vi "密码到期.vi"() -> ()   [LabVIEW 2016]
panel:
  out "密码生效":bool
  out "到期了":bool
  in  "密码输入":string
  in  "停止":bool
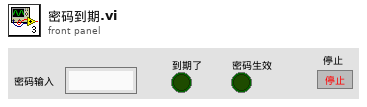
[diagram p1: front panel]
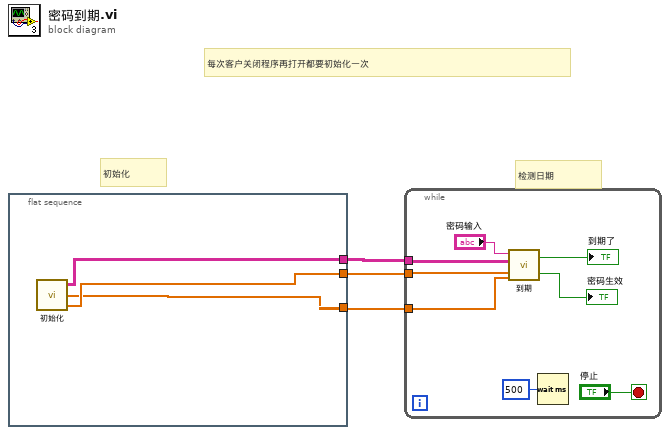
[diagram p0: block diagram]
diagram:
  # "检测日期"
  # "初始化"
  # "每次客户关闭程序再打开都要初始化一次"
  n1 = flat-sequence {
    tunnel: [w5] -> w3
    tunnel: [w6] -> w2
    tunnel: [w4] -> w1
    frame #0 {
      n2 = call "初始化.vi"() -> ("first row"=w5:dbl[], "最终选择的真实日期"=w4:dbl[], "密码"=w6:string[][])  [unwired: 3 in]
    }
  }
  n3 = while {
    tunnel: w3 -> [w8]
    tunnel: w2 -> [w9]
    tunnel: w1 -> [w7]
    stop <- "停止" stop-if-true
    n4 = call "到期.vi"("最终选择的真实的日期"=w7, "加期限后的日期"=w8, "密码和期限"=w9, "密码输入"="密码输入") -> ("密码生效"=→"密码生效":bool, "到期了"=→"到期了":bool)
    n5 = Wait (ms)(milliseconds to wait=u32 500 ("等待时间（毫秒）")) -> ()  [unwired: 1 out]
  }
